vi "MQTTParseTopic.vi"(8 "error in (no error)":errorcluster, 10 "Array":string[](array[string])=["qpd/x", "qpd/y", "qpd/vals", ""], 11 "connection ID":refnum<k5>) -> (0 "error out":errorcluster, 1 "String":string, 2 "Double":dbl, 3 "connection ID out":refnum<k5>, 4 "Message":string="MQIsdp", 5 "Topic Name":string="Topic", 7 "output cluster":T2)   [LabVIEW 2017]
uses:
  <vilib>/daq.io/MQTT LabVIEW Client/Controls/MessageType.ctl
  <vilib>/daq.io/MQTT LabVIEW Client/MQTT_Functions.lvlib
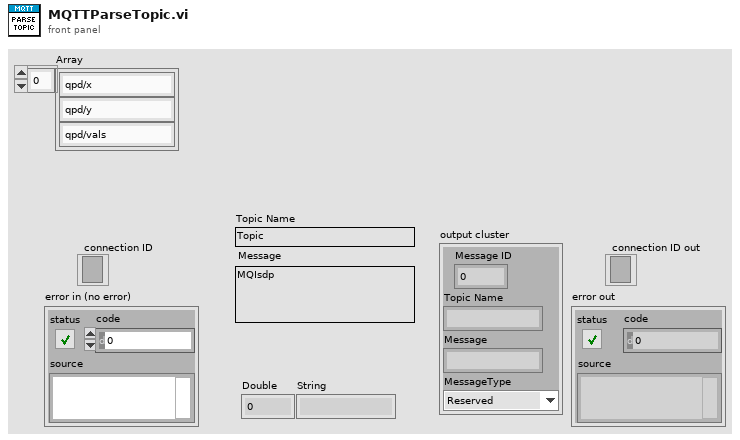
[diagram p1: front panel]
types:
  T1 = typedef "MQTT_Functions.lvlib/MessageType.ctl" = enum32{"Reserved", "CONNECT", "CONNACK", "PUBLISH", "PUBACK", "PUBREC", "PUBREL", "PUBCOMP", "SUBSCRIBE", "SUBACK", "UNSUBSCRIBE", "UNSUBACK", "PINGREQ", "PINGRESP", "DISCONNECT", "Reserved2"}
  T2 = cluster{"Message ID":u16, "Topic Name":string, "Message":string, "MessageType":T1}
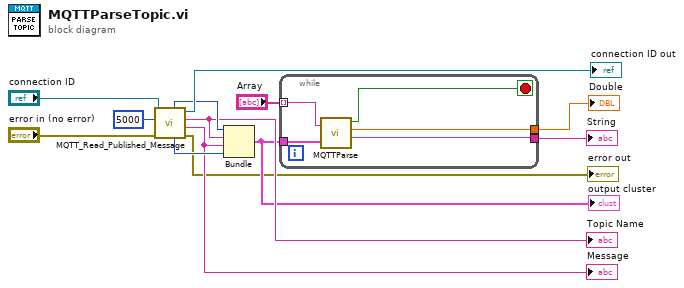
[diagram p0: block diagram]
diagram:
  n1 = call <vilib>:"MQTT_Read_Published_Message.vi"("error in (no error)"="error in (no error)", "Timeout"=5000 ("timeout ms (25000)"), "connection ID"="connection ID") -> ("error out"=→"error out":errorcluster, "Message"=w8:string, "Topic Name"=w9:string, "connection ID out"=→"connection ID out":refnum<k5>, "MessageType"=w11:T1, "Message ID"=w12:u16)  [unwired: 3 in]
  "Topic Name" <- w9
  "Message" <- w8
  n2 = Bundle("Message ID"=w12, "Topic Name"=w9, "Message"=w8, "MessageType"=w11) -> (w7:T2)  [unwired: 1 in]
  "output cluster" <- w7
  n3 = while {
    tunnel: w7 -> [w18]
    tunnel: "Array" -> [w17] mode=indexing
    tunnel: [w15] -> w2
    tunnel: [w14] -> w1
    stop <- w16 stop-if-true
    n4 = call "MQTTParse.vi"("topic"=w17, "Input message"=w18) -> ("Success?"=w16:bool, "Double"=w15:dbl, "String"=w14:string)  [unwired: 3 in]
  }
  "Double" <- w2
  "String" <- w1
